vi "Pre Launch Init.vi"(11 "Transfer Line in":refnum<class "Transfer Line.lvclass">) -> (0 "error out":errorcluster, 3 "Transfer Line out":refnum<class "Transfer Line.lvclass">)   [LabVIEW 2015, in "cRIO-Carbondioxide.lvlib" / "CO2-Actor.lvlib" / "Transfer Line.lvclass"]
doc: "(<B>Filename</B>: Actor Framework.lvlib:Actor.lvclass:Pre Launch Init.vi)\n\nDefines behavior that occurs after the Launch Actor method is invoked but before the actor's Actor Core method begins running.\n\nThe Pre Launch Init method is guaranteed to finish before the Launch Actor method returns to its caller and before the actor itself receives any messages. Any references that the Pre Launch Init method obtains are guaranteed to have the same lifetime as the actor itself. Any errors that the Pre Launch Init method returns will abort the launch.\n\nBy default, this method does nothing. A descendant class may override it to define behavior."
uses:
  Transfer Line.lvclass
  CO2 Actor/CO2 Actor.lvclass
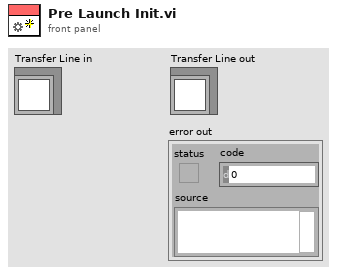
[diagram p1: front panel]
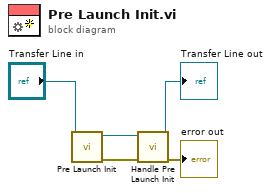
[diagram p0: block diagram]
diagram:
  n1 = call-parent "Pre Launch Init.vi"("CO2 Actor in"="Transfer Line in") -> ("error out"=w5:errorcluster, "CO2 Actor out"=w4:refnum<class "Transfer Line.lvclass">)  [unwired: 9 in]
  n2 = call "Handle Pre Launch Init.vi"("error in (no error)"=w5, "Transfer Line in"=w4) -> ("error out"=→"error out":errorcluster, "Transfer Line out"=→"Transfer Line out":refnum<class "Transfer Line.lvclass">)  [unwired: 8 in]
